vi "SetFlashFlowRateSetpoint.vi"(7 "Timeout (ms)":u32=2000, 8 "Error In":errorcluster, 10 "Setpoint (mL/min)":dbl format="%.1f", 11 "Sierra M100 In":refnum<visa-resource-name>) -> (0 "Error Out":errorcluster, 2 "Set?":bool, 3 "Sierra M100 Out":refnum<visa-resource-name>)   [LabVIEW 2012, in "Sierra-M100.lvlib"]
doc: "This VI sets the flow rate setpoint in the flash memory of the mass flow controller (MFC). The flash memory is non-volatile and will retain the setpoint during power cycling. Use \"Set Flow Rate\" VI instead."
uses:
  Sierra-M100.lvlib
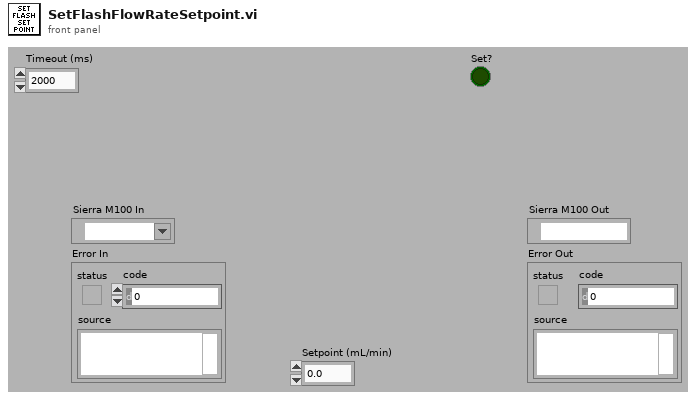
[diagram p1: front panel]
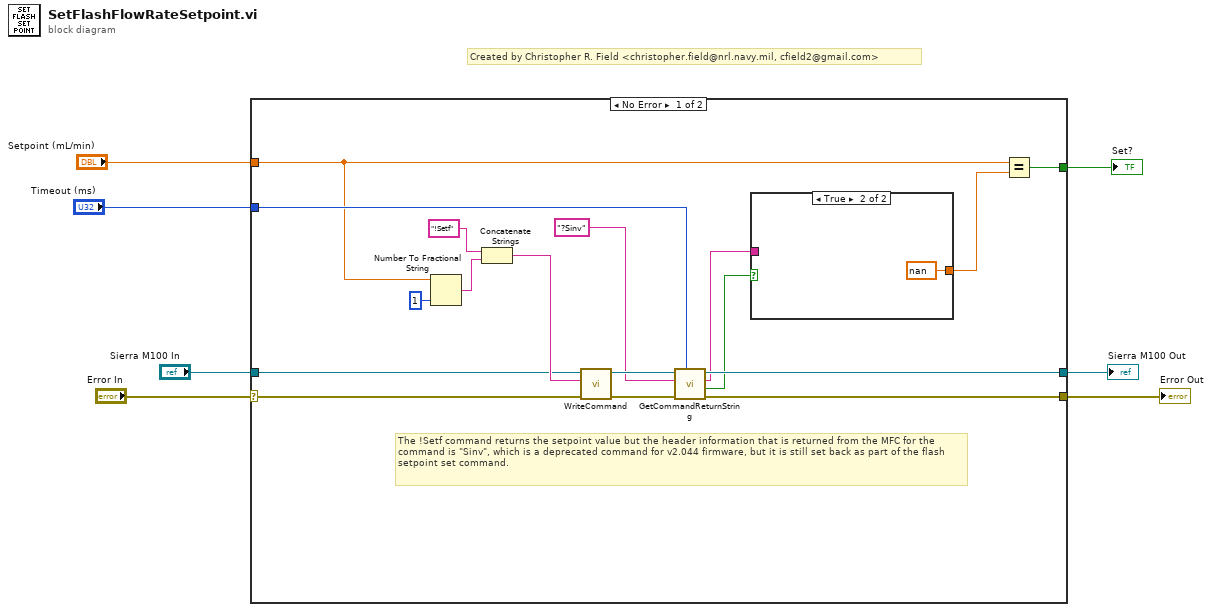
[diagram p0: block diagram]
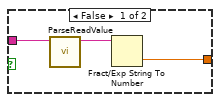
[diagram p2: hidden frame]
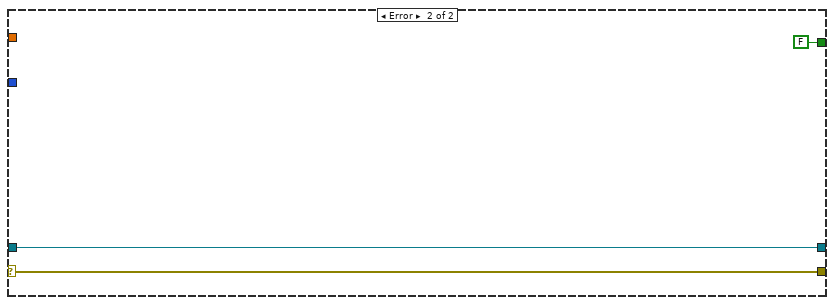
[diagram p3: hidden frame]
diagram:
  # "Created by Christopher R. Field <christopher.field@nrl.navy.mil, cfield2@gmail.com>"
  n1 = case shown="No Error" "Error In" {
    selector: "Error In" -> [w8 w31]
    tunnel: "Sierra M100 In" -> [w21 w30]
    tunnel: "Timeout (ms)" -> [w17 _]
    tunnel: [w15 w30] -> w5
    tunnel: [w14 w31] -> w4
    tunnel: "Setpoint (mL/min)" -> [w11 _]
    tunnel: [w9 FALSE] -> w3
    frame No Error {
      # "The !Setf command returns the setpoint value but the header information that is returned from the MFC for the command is \"Sinv\", which is a deprecated command for v2.044 firmware, but it is still set back as part of the flash setpoint set command."
      n2 = Number To Fractional String(number=w11, precision (6)=i16 1) -> (F-format string=w23:string)  [unwired: 2 in]
      n3 = Concatenate Strings("!Setf", w23) -> (w22:string)
      n4 = call "WriteCommand.vi"("Error In"=w8, "Command"=w22, "Sierra M100 In"=w21) -> ("Error Out"=w18:errorcluster, "Sierra M100 Out"=w19:refnum<visa-resource-name>)  [unwired: 5 in, 2 out]
      n5 = call "GetCommandReturnString.vi"("Timeout (ms)"=w17, "Error In"=w18, "Command"="?Sinv", "Sierra M100 In"=w19) -> ("Error Out"=w14:errorcluster, "Timeout?"=w12:bool, "Return String"=w13:string, "Sierra M100 Out"=w15:refnum<visa-resource-name>)  [unwired: 4 in]
      n6 = case shown="True" w12 {
        tunnel: w13 -> [w27 _]
        tunnel: [w25 nan] -> w10
        frame False {
          n7 = call "ParseReadValue.vi"("Read Buffer"=w27) -> ("Value"=w26:string)  [unwired: 10 in]
          n8 = Fract/Exp String To Number(string=w26) -> (number=w25:dbl)  [unwired: 3 in, 1 out]
        }
        frame True {
        }
      }
      n9 = Equal?(x=w11, y=w10) -> (x = y?=w9:bool)
    }
    frame Error {
    }
  }
  "Sierra M100 Out" <- w5
  "Error Out" <- w4
  "Set?" <- w3
